vi "Motor with Encoder - Bang Bang DrH.vi"() -> ()   [LabVIEW 2016]
doc: "This example shows how to move a motor connected to an encoder and a wheel, and then read information about the system from an encoder.\n\nThis is an example of how to use feedback (from the encoder) to create an open loop system. If some control method was used, for example using PID, a closed loop system could be created.\n\nThis example expects a USB cable connected from your development PC to the Type B USB Jack (next to the power input) on the roboRIO.\n\nThis example requires the Driver Station to be running with Teleoperated Enabled."
uses:
  <vilib>/Rock Robotics/SystemInterfaces/DIO/FPGA_DIOChannel.ctl
  <vilib>/Rock Robotics/WPI/Encoder/WPI_EncoderType.ctl
  <vilib>/Rock Robotics/SystemInterfaces/DIO/FPGA_DIOPWMChannel.ctl
  <vilib>/Rock Robotics/WPI/Counter/WPI_CounterDigitalInputToDigitalSource.vi
  <vilib>/Rock Robotics/WPI/MotorControl/WPI_MotorControlOpen SPARK.vi
  <vilib>/gmath/NI_Gmath.lvlib
panel:
  in  "Update":bool
  in  "lower limit":dbl=-100.0 format="%#_13g"
  in  "upper limit":dbl=100.0 format="%#_13g"
  out "Error":dbl(graph)
  out "Error":dbl
  out "DS Original":dbl
  in  "Neg Drive Signal":dbl=0.5
  in  "Pos Drive Signal":dbl=1.0
  in  "Target RPM":dbl
  in  "milliseconds to wait":u32=10
  out "Loop Time (s)":dbl format="%_6f"
  out "RPM":dbl=1324.567
  out "XY Graph":cluster{dbl[], dbl[]}[](graph)
  out "Waveform Chart":dbl(graph)
  in  "Motor PWM Channel":T1=enum."PWM 9"
  in  "Number Samples to Average":u8=1 min=1 max=128
  in  "Invert Direction":bool=TRUE
  in  "Decoding Type":T2=enum."4x"
  in  "DistancePerCount (deg)":dbl=0.351563
  in  "Encoder B Channel":T3=enum."DIO 1"
  in  "Encoder A Channel":T3
  in  "Minimum Rate":dbl=20.0
  in  "Stop":bool
  out "Encoder Alarm Status":string="Encoder Stopped"
  out "Encoder Direction":string="Forward"
  # "These can be set while running."
  # "Output information."
  # "Set these inputs before running."
  # "This example requires the Driver Station to be running with Teleoperated Enabled."
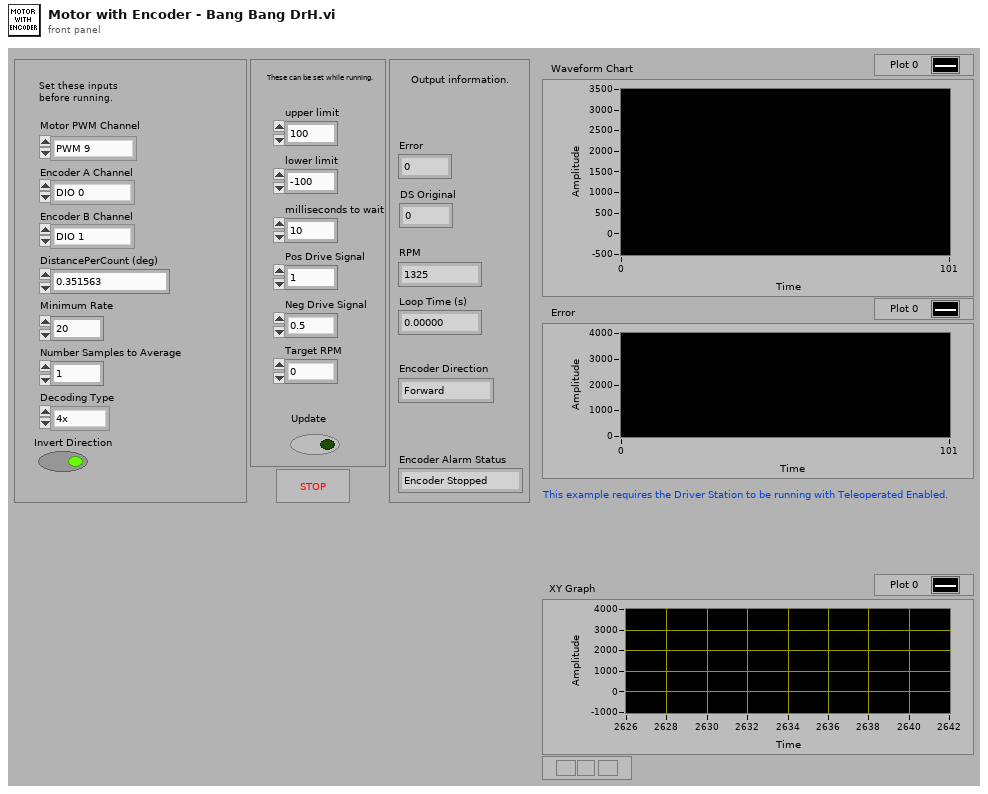
[diagram p1: front panel]
types:
  T1 = typedef "FPGA_DIOPWMChannel.ctl" = enum8{"PWM 0", "PWM 1", "PWM 2", "PWM 3", "PWM 4", "PWM 5", "PWM 6", "PWM 7", "PWM 8", "PWM 9", "PWM MXP 0", "PWM MXP 1", "PWM MXP 2", "PWM MXP 3", "PWM MXP 4", "PWM MXP 5", "PWM MXP 6", "PWM MXP 7", "PWM MXP 8", "PWM MXP 9", "Invalid"}
  T2 = typedef "WPI_EncoderType.ctl" = enum16{"1x", "2x", "4x"}
  T3 = typedef "FPGA_DIOChannel.ctl" = enum8{"DIO 0", "DIO 1", "DIO 2", "DIO 3", "DIO 4", "DIO 5", "DIO 6", "DIO 7", "DIO 8", "DIO 9", "DIO MXP 0", "DIO MXP 1", "DIO MXP 2", "DIO MXP 3", "DIO MXP 4", "DIO MXP 5", "DIO MXP 6", "DIO MXP 7", "DIO MXP 8", "DIO MXP 9", "DIO MXP 10", "DIO MXP 11", "DIO MXP 12", "DIO MXP 13", "DIO MXP 14", "DIO MXP 15", "SPI Port CS1", "SPI Port CS2", "SPI Port CS3", "SPI Port MISO", "SPI Port MOSI", "Invalid"}
  T4 = typedef "WPI_MotorControlDeviceRef.ctl" = cluster{"DeviceStatus":errorcluster, "Type":T5, "PWM":cluster{"PWM Channel":T1, "DeadBand":T6}, "CAN":cluster{"Device Number":u8, "SetOutput VI Ref":variant, "GetOutput VI Ref":variant, "Enable VI Ref":variant, "Disable VI Ref":variant, "Data":variant}, "Invert":bool}
  T5 = typedef "WPI_MotorControlType.ctl" = enum16{"PWM", "CAN"}
  T6 = typedef "WPI_PWMDeadband.ctl" = cluster{"Name":string, "maxPositivePwm":i32, "minPositivePwm":i32, "centerPwm":i32, "maxNegativePwm":i32, "minNegativePwm":i32, "angularRange":u16}
  T7 = typedef "WPI_DigitalInputDevRef.ctl" = cluster{"DevStatus":errorcluster, "DIO Channel":T3}
  T8 = typedef "FPGA_CounterEncoderSourceConvertionLVSourceType.ctl" = cluster{"DevStatus":errorcluster, "AnalogTriggerMode?":bool, "DigitalMode":cluster{"DIO Channel":T9}, "AnalogTriggerMode":cluster{"AnalogTriggerIndex":T10, "OutputType":T11}}
  T9 = typedef "FPGA_DIODigitalSourceChannel.ctl" = enum8{"DIO 0", "DIO 1", "DIO 2", "DIO 3", "DIO 4", "DIO 5", "DIO 6", "DIO 7", "DIO 8", "DIO 9", "DIO MXP 0", "DIO MXP 1", "DIO MXP 2", "DIO MXP 3", "DIO MXP 4", "DIO MXP 5", "DIO MXP 6", "DIO MXP 7", "DIO MXP 8", "DIO MXP 9", "DIO MXP 10", "DIO MXP 11", "DIO MXP 12", "DIO MXP 13", "DIO MXP 14", "DIO MXP 15", "Disabled"}
  T10 = typedef "FPGA_AnalogTriggerIndex.ctl" = enum8{"Trig 0", "Trig 1", "Trig 2", "Trig 3", "Trig 4", "Trig 5", "Trig 6", "Trig 7", "Invalid"}
  T11 = typedef "FPGA_AnalogTriggerOutType.ctl" = enum16{"InWindow", "TriggerState", "Rising", "Falling"}
  T12 = typedef "WPI_EncoderDevRef.ctl" = cluster{"DevStatus":errorcluster, "EncoderIndex":T13, "CounterIndex":T14, "DistancePerCount":dbl, "Decoding Type":T2}
  T13 = typedef "FPGA_EncoderIdx.ctl" = enum8{"Enc 0", "Enc 1", "Enc 2", "Enc 3", "Enc 4", "Enc 5", "Enc 6", "Enc 7", "Invalid"}
  T14 = typedef "FPGA_CounterCtrSystemIndex.ctl" = enum8{"Ctr 0", "Ctr 1", "Ctr 2", "Ctr 3", "Ctr 4", "Ctr 5", "Ctr 6", "Ctr 7", "Invalid"}
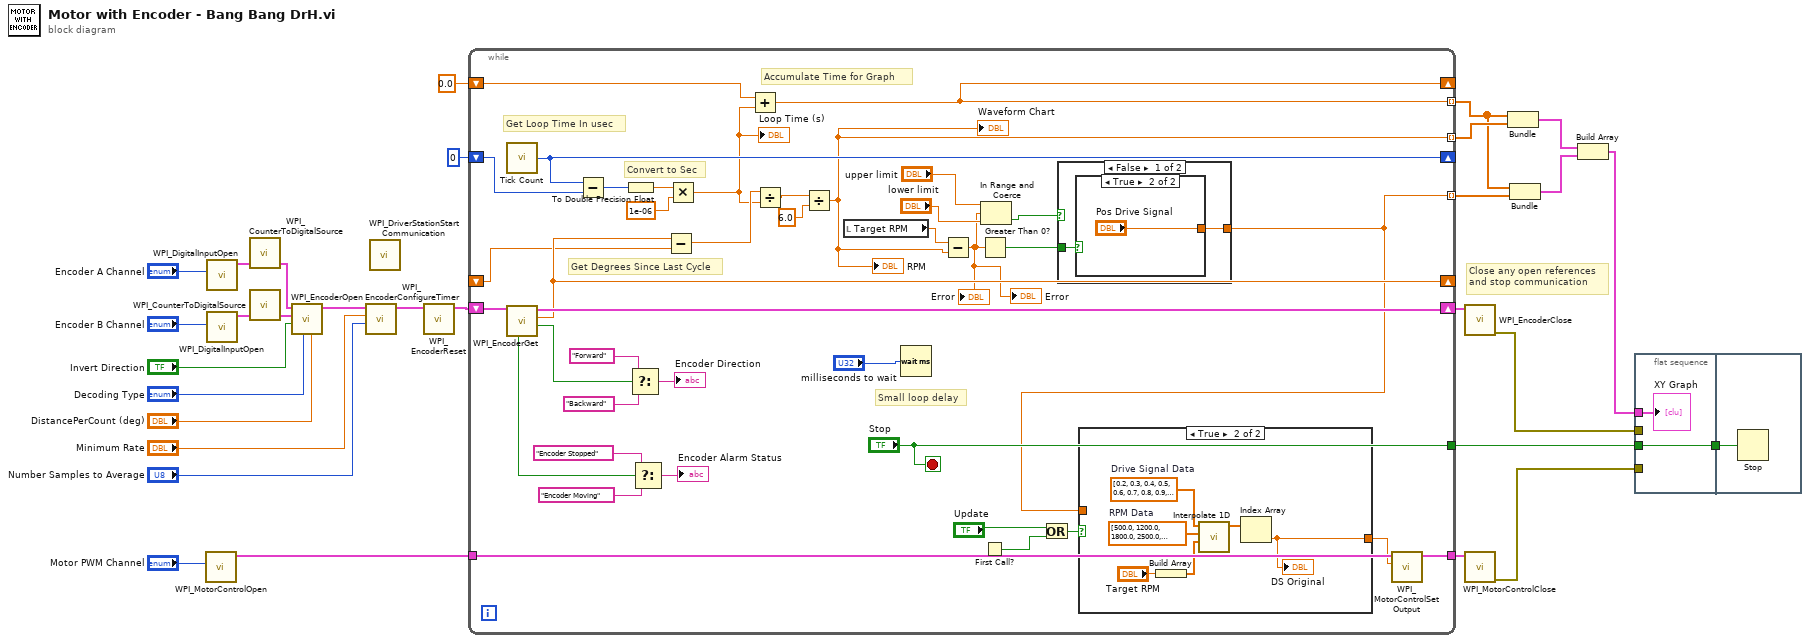
[diagram p0: block diagram]
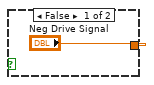
[diagram p3: hidden frame]
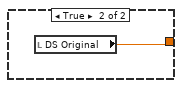
[diagram p4: hidden frame]
diagram:
  # "Close any open references\nand stop communication"
  n1 = call-poly <vilib>:"WPI_MotorControlOpen.vi"("PWM Channel"="Motor PWM Channel") -> ("MotorControlDeviceRef"=w1:T4)  [unwired: 3 in, 7 out]
  n2 = call <vilib>:"WPI_DigitalInputOpen.vi"("DIO Channel"="Encoder A Channel") -> ("DigitalInputDevRef"=w27:T7)  [unwired: 1 in, 9 out]
  n3 = call <vilib>:"WPI_DigitalInputOpen.vi"("DIO Channel"="Encoder B Channel") -> ("DigitalInputDevRef"=w28:T7)  [unwired: 1 in, 9 out]
  n4 = call-poly <vilib>:"WPI_CounterToDigitalSource.vi"("DigitalInputDevRef"=w27) -> ("Digital Source"=w26:T8)  [unwired: 6 out]
  n5 = call-poly <vilib>:"WPI_CounterToDigitalSource.vi"("DigitalInputDevRef"=w28) -> ("Digital Source"=w29:T8)  [unwired: 6 out]
  n6 = call <vilib>:"WPI_EncoderOpen.vi"("DistancePerCount"="DistancePerCount (deg)", "Decoding Type"="Decoding Type", "Invert Direction (False)"="Invert Direction", "BSource"=w29, "ASource"=w26) -> ("EncoderDevRef"=w20:T12)  [unwired: 3 in, 3 out]
  n7 = call <vilib>:"WPI_EncoderConfigureTimer.vi"("Number Samples to Average"="Number Samples to Average", "Minimum Rate"="Minimum Rate", "EncoderDevRef"=w20) -> ("EncoderDevRef"=w13:T12)  [unwired: 1 in, 7 out]
  n8 = call <vilib>:"WPI_DriverStationStart Communication.vi"() -> ()  [unwired: 2 in, 10 out]
  n9 = call <vilib>:"WPI_EncoderReset.vi"("EncoderDevRef"=w13) -> ("EncoderDevRef"=w12:T12)  [unwired: 1 in, 9 out]
  n10 = while {
    shift-right: [w55] -> w30
    shift-left: w12 -> [w58]
    tunnel: ["Stop"] -> w15
    tunnel: w1 -> [w61]
    tunnel: [w60] -> w17
    tunnel: [w41] -> w14 mode=indexing
    tunnel: [w43] -> w8 mode=indexing
    shift-right: [w54] -> _
    shift-left: u32 0 ("Tick Count(uSec)") -> [w53]
    shift-right: [w52] -> _
    shift-left: _ -> [w51]
    shift-right: [w43] -> _
    shift-left: 0.0 ("Tick Count(uSec)") -> [w44]
    tunnel: [w35] -> w7 mode=indexing
    stop <- "Stop" stop-if-true
    # "Accumulate Time for Graph"
    # "Get Degrees Since Last Cycle"
    # "Convert to Sec"
    # "Get Loop Time In usec"
    # "Small loop delay"
    n11 = call "Tick Count"() -> ("Tick Count(uSec)"=w54:u32)
    n12 = call <vilib>:"WPI_EncoderGet.vi"("EncoderDevRef"=w58) -> ("Direction"=w67:bool, "Distance"=w52:dbl, "EncoderDevRef"=w55:T12, "Stopped"=w66:bool)  [unwired: 1 in, 6 out]
    n13 = Subtract(x=w54, y=w53) -> (x-y=w50:u32)
    n14 = To Double Precision Float(number=w50) -> (double precision float=w48:dbl)
    n15 = Select(t="Forward", s=w67, f="Backward") -> (s? t:f=→"Encoder Direction":string)
    n16 = Select(t="Encoder Stopped", s=w66, f="Encoder Moving") -> (s? t:f=→"Encoder Alarm Status":string)
    n17 = Subtract(x=w52, y=w51) -> (x-y=w47:dbl)
    n18 = Multiply(x=w48, y=1e-06) -> (x*y=w45:dbl)
    "Loop Time (s)" <- w45
    n19 = Add(x=w44, y=w45) -> (x+y=w43:dbl)
    n20 = Divide(x=w47, y=w45) -> (x/y=w46:dbl)
    n21 = Divide(x=w46, y=6.0) -> (x/y=w41:dbl)
    "Waveform Chart" <- w41
    "RPM" <- w41
    n22 = local read "Target RPM"() -> (w42:dbl)
    n23 = Wait (ms)(milliseconds to wait="milliseconds to wait") -> ()  [unwired: 1 out]
    n24 = Subtract(x=w42, y=w41) -> (x-y=w37:dbl)
    "Error" <- w37
    "Error" <- w37
    n25 = Greater Than 0?(x=w37) -> (x > 0?=w40:bool)
    n26 = First Call?() -> (First Call?: T/F=w31:bool)
    n27 = In Range and Coerce(upper limit="upper limit", x=w37, lower limit="lower limit") -> (In Range?=w36:bool)  [unwired: 1 out]
    n28 = Or(x="Update", y=w31) -> (x .or. y?=w32:bool)
    n29 = case shown="False" w36 {
      tunnel: w40 -> [w78 _]
      tunnel: [w77 w81] -> w35
      frame False {
        n30 = case shown="True" w78 {
          tunnel: ["Neg Drive Signal" "Pos Drive Signal"] -> w77
          frame False {
          }
          frame True {
          }
        }
      }
      frame True {
        n31 = local read "DS Original"() -> (w81:dbl)
      }
    }
    n32 = case shown="True" w32 {
      tunnel: [w70 w71] -> w34
      tunnel: w35 -> [w70 _]
      frame False {
      }
      frame True {
        w76 = dbl[] [500.0, 1200.0, 1800.0, 2500.0, 3200.0, 3800.0, 4400.0, 4900.0, 5400.0]  # RPM Data
        w75 = dbl[] [0.2, 0.3, 0.4, 0.5, 0.6, 0.7, 0.8, 0.9, 1.0]  # Drive Signal Data
        n33 = Build Array("Target RPM") -> (w73:dbl[])
        n34 = call <vilib>:"Interpolate 1D.vi"("xi"=w73, "X"=w76, "Y"=w75) -> ("yi"=w72:dbl[])  [unwired: 6 in, 2 out]
        n35 = Index Array(array=w72) -> (element=w71:dbl)  [unwired: 1 in]
        "DS Original" <- w71
      }
    }
    n36 = call <vilib>:"WPI_MotorControlSetOutput.vi"("Output"=w34, "MotorControlDevRef"=w61) -> ("MotorControlDevRef"=w60:T4)  [unwired: 2 in, 7 out]
  }
  n37 = call <vilib>:"WPI_EncoderClose.vi"("EncoderDevRef"=w30) -> ("error out"=w3:errorcluster)  [unwired: 2 in, 8 out]
  n38 = call <vilib>:"WPI_MotorControlClose.vi"("MotorControlDevRef"=w17) -> ("error out"=w2:errorcluster)  [unwired: 1 in, 9 out]
  n39 = Bundle(w8, w14) -> (w6:cluster{dbl[], dbl[]})  [unwired: 1 in]
  n40 = Bundle(w8, w7) -> (w5:cluster{dbl[], dbl[]})  [unwired: 1 in]
  n41 = Build Array(w6, w5) -> (w4:cluster{dbl[], dbl[]}[])
  n42 = flat-sequence {
    tunnel: w15 -> [w83]
    tunnel: [w83] -> w11
    tunnel: w4 -> [w82]
    tunnel: w3 -> [_]
    tunnel: w2 -> [_]
    tunnel: w11 -> [w84]
    frame #0 {
      "XY Graph" <- w82
    }
    frame #1 {
      n43 = Stop(stop? (T)=w84) -> ()
    }
  }
